vi "Error handler RT.vi"(8 "error in":errorcluster, 11 "Message Queue":refnum<queue>) -> (0 "error out":errorcluster, 3 "Duq Message Queue":refnum<queue>)   [LabVIEW 2022 SP3]
uses:
  c8e64d7e-ce45-4cfd-9636-85734d5256d9.vi
  6ecc959c-78fe-438c-aec5-e12e03fb8790.vi
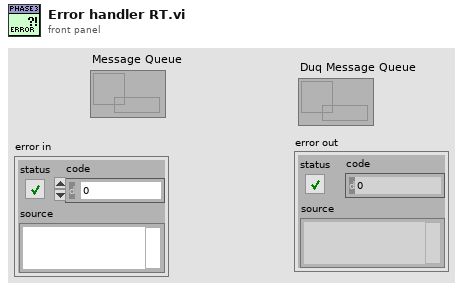
[diagram p1: front panel]
types:
  T1 = cluster{"Error Code":string, "Error Source":string}
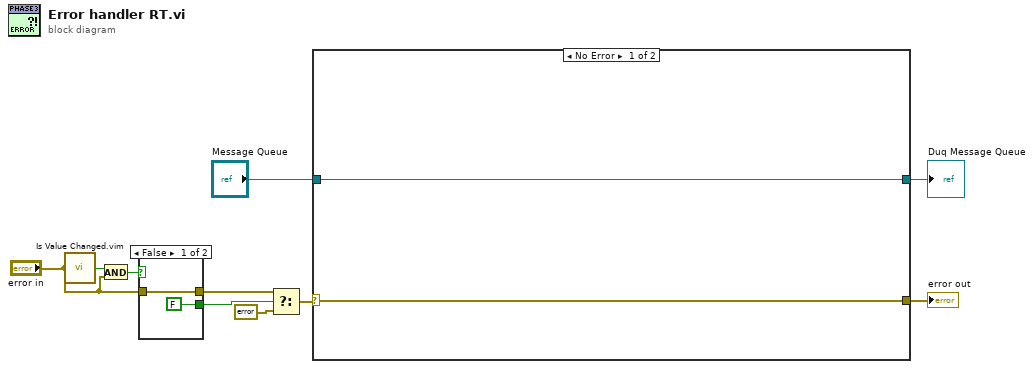
[diagram p0: block diagram]
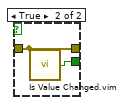
[diagram p2: hidden frame]
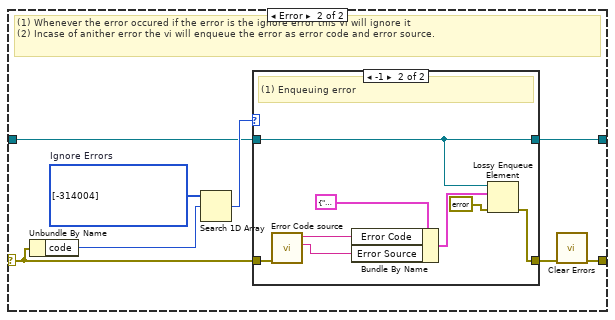
[diagram p3: hidden frame]
diagram:
  n1 = call "Is Value Changed.vim"("value"="error in") -> ("changed or first call?"=w7:bool)
  n2 = And(x=w7, y="error in") -> (x .and. y?=w3:bool)
  n3 = case shown="False" w3 {
    tunnel: "error in" -> [w11 w13]
    tunnel: [FALSE ("changed or first call?") w14] -> w5
    tunnel: [w11 w13] -> w4
    frame False {
    }
    frame True {
      n4 = call "Is Value Changed.vim"("value"=w13) -> ("changed or first call?"=w14:bool)
    }
  }
  n5 = Select(t=w4, s=w5, f=errorcluster {"status"=FALSE, "code"=0, "source"=""}) -> (s? t:f=w8:errorcluster)
  n6 = case shown="No Error" w8 {
    selector: w8 -> [w16 w21]
    tunnel: [w16 w19] -> w10
    tunnel: "Message Queue" -> [w15 w17]
    tunnel: [w15 w18] -> w1
    frame No Error {
    }
    frame Error {
      w23 = i32[] [-314004]  # Ignore Errors
      # "(1) Whenever the error occured if the error is the ignore error this Vi will ignore it\n(2) Incase of anither error the vi will enqueue the error as error code and error source."
      n7 = Unbundle By Name(w21) -> ("code"=w24:i32)
      n8 = Search 1D Array(1D array=w23, element=w24) -> (index of element=w22:i32)  [unwired: 1 in]
      n9 = case shown="-1" w22 {
        tunnel: w21 -> [w26 w30]
        tunnel: [w26 w32] -> w20
        tunnel: w17 -> [w25 w27]
        tunnel: [w25 w27] -> w18
        frame 0, Default {
        }
        frame -1 {
          # "(1) Enqueuing error"
          n10 = call "Error Code source .vi"("error in (no error)"=w30) -> ("String"=w28:string, "String 2"=w29:string)  [unwired: 9 in]
          n11 = Bundle By Name(cluster=T1 {"Error Code"="", "Error Source"=""} ("element"), "Error Code"=w29, "Error Source"=w28) -> (w33:T1)
          n12 = Lossy Enqueue Element(queue=w27, element=w33, error in (no error)=errorcluster {"status"=FALSE, "code"=0, "source"=""}) -> (error out=w32:errorcluster)  [unwired: 3 out]
        }
      }
      n13 = call <vilib>:"Clear Errors.vi"("error in (no error)"=w20) -> ("error out"=w19:errorcluster)  [unwired: 5 in, 1 out]
    }
  }
  "error out" <- w10
  "Duq Message Queue" <- w1
